vi "LVdouble connection.vi"() -> ()   [LabVIEW 2019]
doc: "This example performs a serial port write and a serial port read. The parameters set for the serial port must match the parameters of the connected instrument or device. The VISA Configure Serial Port VI sets the configuration parameters. The front panel displays the controls used to configure the basic parameters, such as baud rate, data bits, and parity. The VI passes the VISA resource name to other VIs that perform operations on that VISA resource. The VISA Write function sends a command to the serial device and the VISA Read function returns data based on the command. The VISA Close function then closes the reference to the serial device. It is important to close the reference; otherwise, further communication through that port might not be possible."
uses:
  Serial - Settings.ctl
  <vilib>/Utility/file.llb/Read Delimited Spreadsheet (DBL).vi
  <vilib>/Instr/_visa.llb/VISA Configure Serial Port (Instr).vi
panel:
  in  "Nominal Load Motor Torque":dbl=198.0
  out "Error Out":errorcluster={"status"=FALSE, "code"=1073676294, "source"="Event Code: 1073676294\r\nVISA Read in Read_Speed_Ref_1_21200.vi->LVdouble connection.vi\r\n-----------------------------------\nEvent Code: 1073676294\r\nVISA Read in Read_torque_Ref_1_21200.vi->LVdouble connection.vi\r\n-----------------------------------\n"}
  out "speed of the car km/h":dbl(knob)=0.002696450428155059 scale=0.0..10.0
  out "Execution time":u32(graph)=1000
  out "x-y 2":sgl
  out "String out":string
  out "read buffer 13":string
  out "read buffer 12":string
  out "read buffer 11":string
  out "read buffer 10":string
  out "read buffer 9":string
  out "read buffer 8":string
  out "read buffer 7":string
  out "Torque_Ref_readings":sgl(graph)
  in  "test_torque_setpoints":path=path "C:/Users/arda/Documents/GitHub/labviewtestbench/torque sp/simplified.txt"
  out "Power(kW)_PMSM":sgl(graph)=-5.360817e-06
  out "I_D":sgl(graph)=-0.16567513
  out "I_Q":sgl(graph)=-0.5964305
  out "I_PMSM":sgl(graph)
  out "Estimated Torque_PMSM":sgl(graph)=-0.5964305
  out "Read RPM-PMSM":dbl(graph)=-0.02861022762954235
  in  "data logging":bool=TRUE
  out "Serial Settings:Wire Mode 2":i8(ring)=-128 items=["Unknown"=-1, "RS485/Wire4"=0, "RS485/Wire2-EchoDTR"=1, "RS485/Wire2-CtrlDTR"=2, "RS485/Wire2-Auto"=3, "RS232/DTE"=-128, "RS232/DCE"=-127, "RS232/Auto"=-126]
  in  "timeout (10sec) 2":u32=10000
  in  "Enable Termination\nChar (T) 2":bool
  in  "Serial Settings 2":T1={"baud rate"=38400, "data bits"=8, "parity"=enum."Even", "stop bits"=10, "flow control"=0} {"flow control" items=["None"=0, "XON/XOFF"=1, "RTS/CTS"=2, "DTR/DSR"=4]; "stop bits" items=["1.0"=10, "1.5"=15, "2.0"=20]; "data bits" min=5 max=8 step=1; "baud rate" items=["75"=75, "110"=110, "134"=134, "150"=150, "300"=300, "600"=600, "1200"=1200, "1800"=1800, "2400"=2400, "4800"=4800, "9600"=7200, "19600"=9600, "14400"=14400, "19200"=19200, "28800"=28800, "38400"=38400, "56000"=56000, "57600"=57600, "115200"=115200, "128000"=128000, "230400"=230400]}
  in  "Hub Motor":refnum<visa-resource-name>="COM4"
  out "Torque Setpoints":dbl(graph)=4.4291015078268256e-09
  in  "Name your log file:":string="24_01_2020_low_cycle_100sec_on_inductionmotor"
  out "Speed Reference":sgl(graph)
  out "Speed Ref in 21202":string
  out "Floating Point 5":sgl
  out "Speed Ref in 21201":string
  in  "write buffer 5":string="\u0002\u0003RÑ\u0000\u0002„¹"
  out "Floating Point 4":sgl
  out "Speed Ref in 21201":string
  in  "write buffer 4":string="\u0002\u0003RÐ\u0000\u0002Õy"
  in  "write buffer 3":string="\u0002\u0003I<\u0000\u0002\u0012h"
  out "read buffer 6":string
  out "read buffer 5":string
  out "read buffer 4":string
  out "read buffer 3":string
  out "read buffer 2":string
  out "read buffer":string
  in  "write buffer 2":string="\u0002\u0003RÏ\u0000\u0002ä¿"
  in  "write buffer":string="\u0002\u0010RÏ\u0000\u0002\u0004\u0000\u0000@ d "
  out "Answer to Write Command":string
  out "Floating Point 3":sgl=5.00679
  out "Speed Ref in 21200":string
  out "Floating Point 2":sgl=0.14305113
  out "Speed Ref in Monitor":string
  out "I_D_IM":sgl(graph)=100.81332
  out "I_q_IM":sgl(graph)=-0.8283757
  out "Power(kW)_IM":sgl(graph)=-0.00012096913
  out "Current(I)_IM":sgl(graph)=100.730484
  in  "RPM and time setpoint file":path=path "C:/Users/arda/Documents/GitHub/labviewtestbench/RPM_setpointfile/ramp(1hz)_lowcycle.txt"
  in  "Tyre Diameter(m)":sgl=0.5
  out "Measured RPM_IM":sgl(graph)=0.028610228
  in  "Enum":T2(ring)=enum."Default"
  in  "Continuous Connection(Def:ON)":bool=TRUE
  out "Estimated Torque_IM":sgl(graph)=-4.347938
  in  "Finish session(Def:Off/False)":bool
  in  "Connectivity Check (Def:Off)":bool
  in  "timeout (10sec)":u32=10000
  out "connection check":u8[](array[numeric])=[0, 0, 0, 2]
  in  "Enable Termination\nChar (T)":bool
  in  "connection_verification":string="\u0002\u0003Fm\u0000\u0002@­"
  out "Serial Settings:Wire Mode":i8(ring)=-128 items=["Unknown"=-1, "RS485/Wire4"=0, "RS485/Wire2-EchoDTR"=1, "RS485/Wire2-CtrlDTR"=2, "RS485/Wire2-Auto"=3, "RS232/DTE"=-128, "RS232/DCE"=-127, "RS232/Auto"=-126]
  in  "Serial Settings":T1={"baud rate"=38400, "data bits"=8, "parity"=enum."Even", "stop bits"=10, "flow control"=0} {"flow control" items=["None"=0, "XON/XOFF"=1, "RTS/CTS"=2, "DTR/DSR"=4]; "stop bits" items=["1.0"=10, "1.5"=15, "2.0"=20]; "data bits" min=5 max=8 step=1; "baud rate" items=["75"=75, "110"=110, "134"=134, "150"=150, "300"=300, "600"=600, "1200"=1200, "1800"=1800, "2400"=2400, "4800"=4800, "9600"=7200, "19600"=9600, "14400"=14400, "19200"=19200, "28800"=28800, "38400"=38400, "56000"=56000, "57600"=57600, "115200"=115200, "128000"=128000, "230400"=230400]}
  in  "Induction Motor":refnum<visa-resource-name>="COM3"
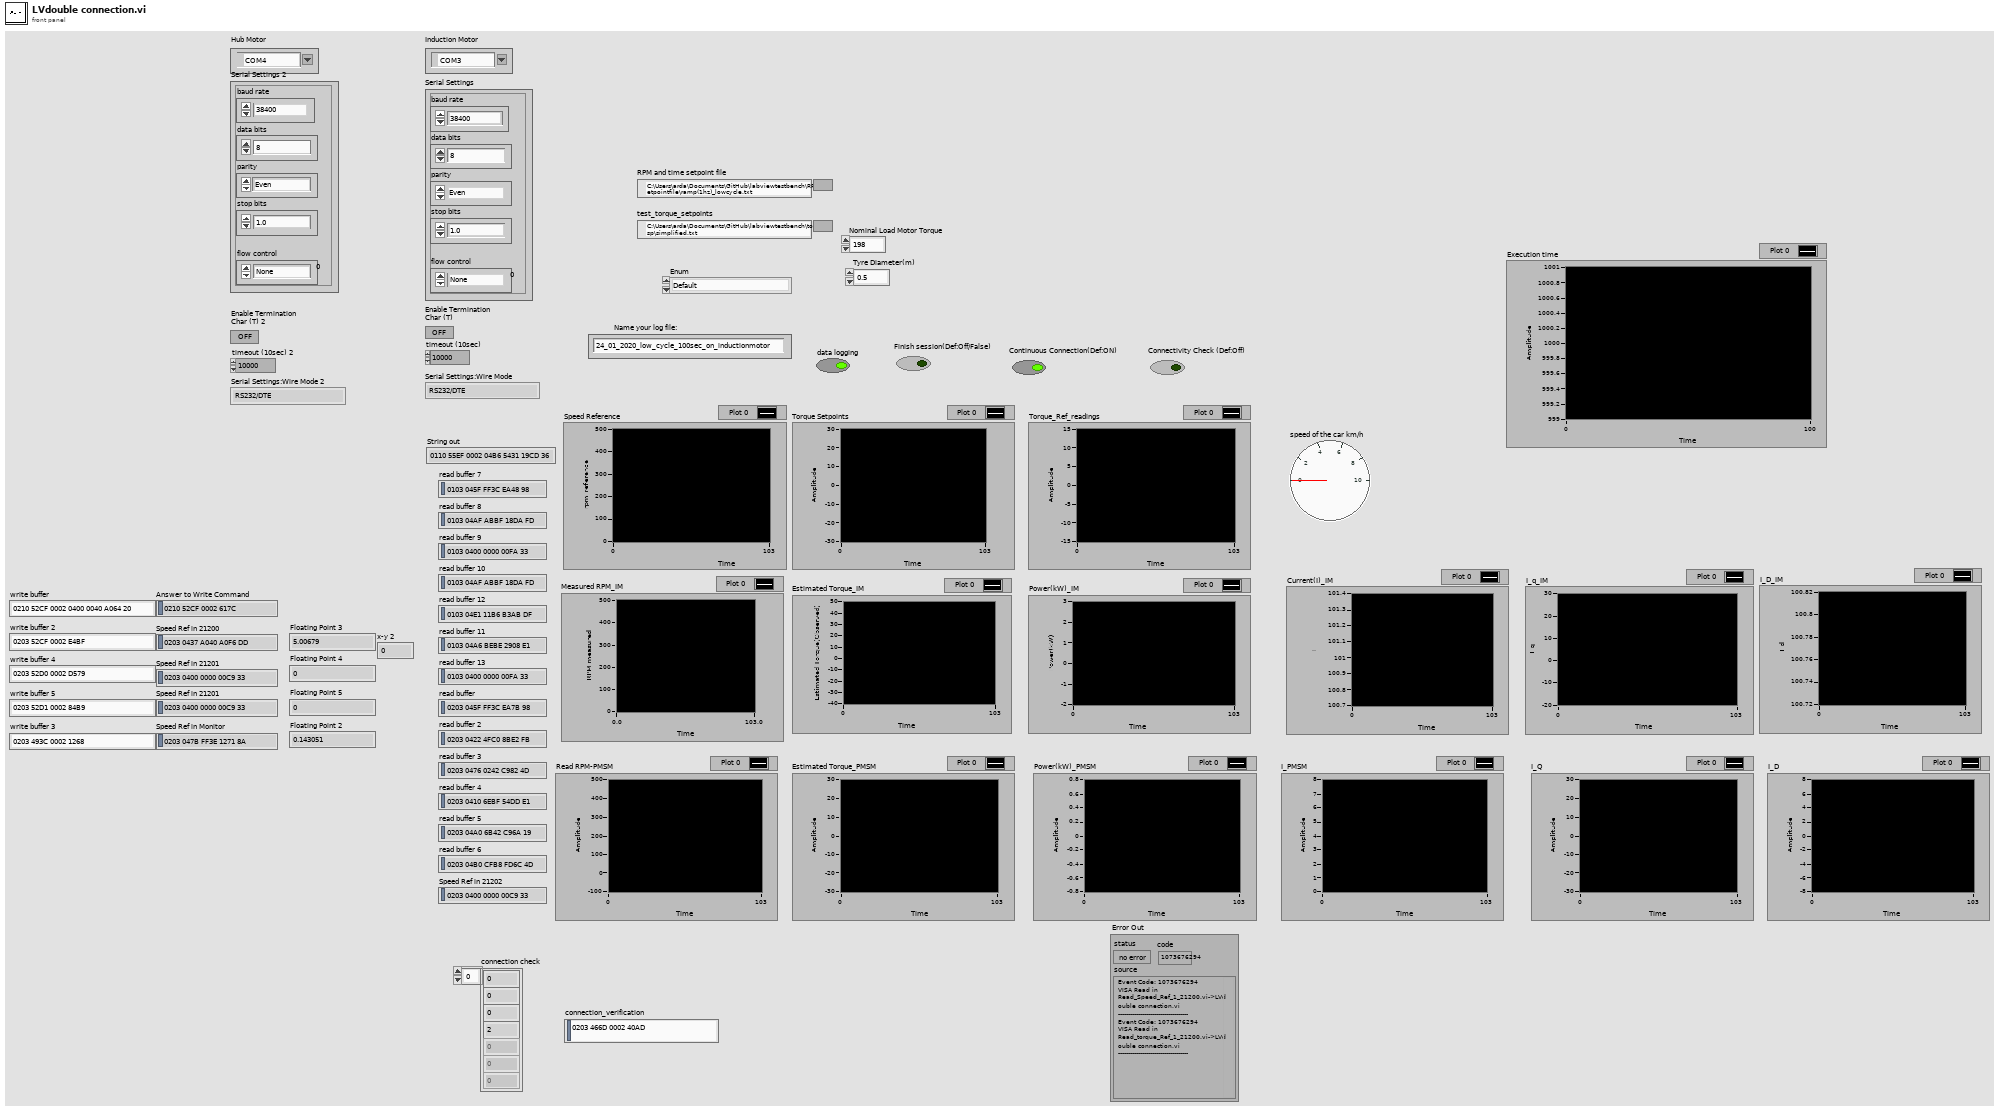
[diagram p1: front panel]
types:
  T1 = typedef "Serial - Settings.ctl" = cluster{"baud rate":u32, "data bits":u16, "parity":enum16{"None", "Odd", "Even", "Mark", "Space"}, "stop bits":u16, "flow control":u16}
  T2 = enum16{"Single Signal Trials", "Default", "Alarm Reset", "Write Save Command", "Drive Reset"}
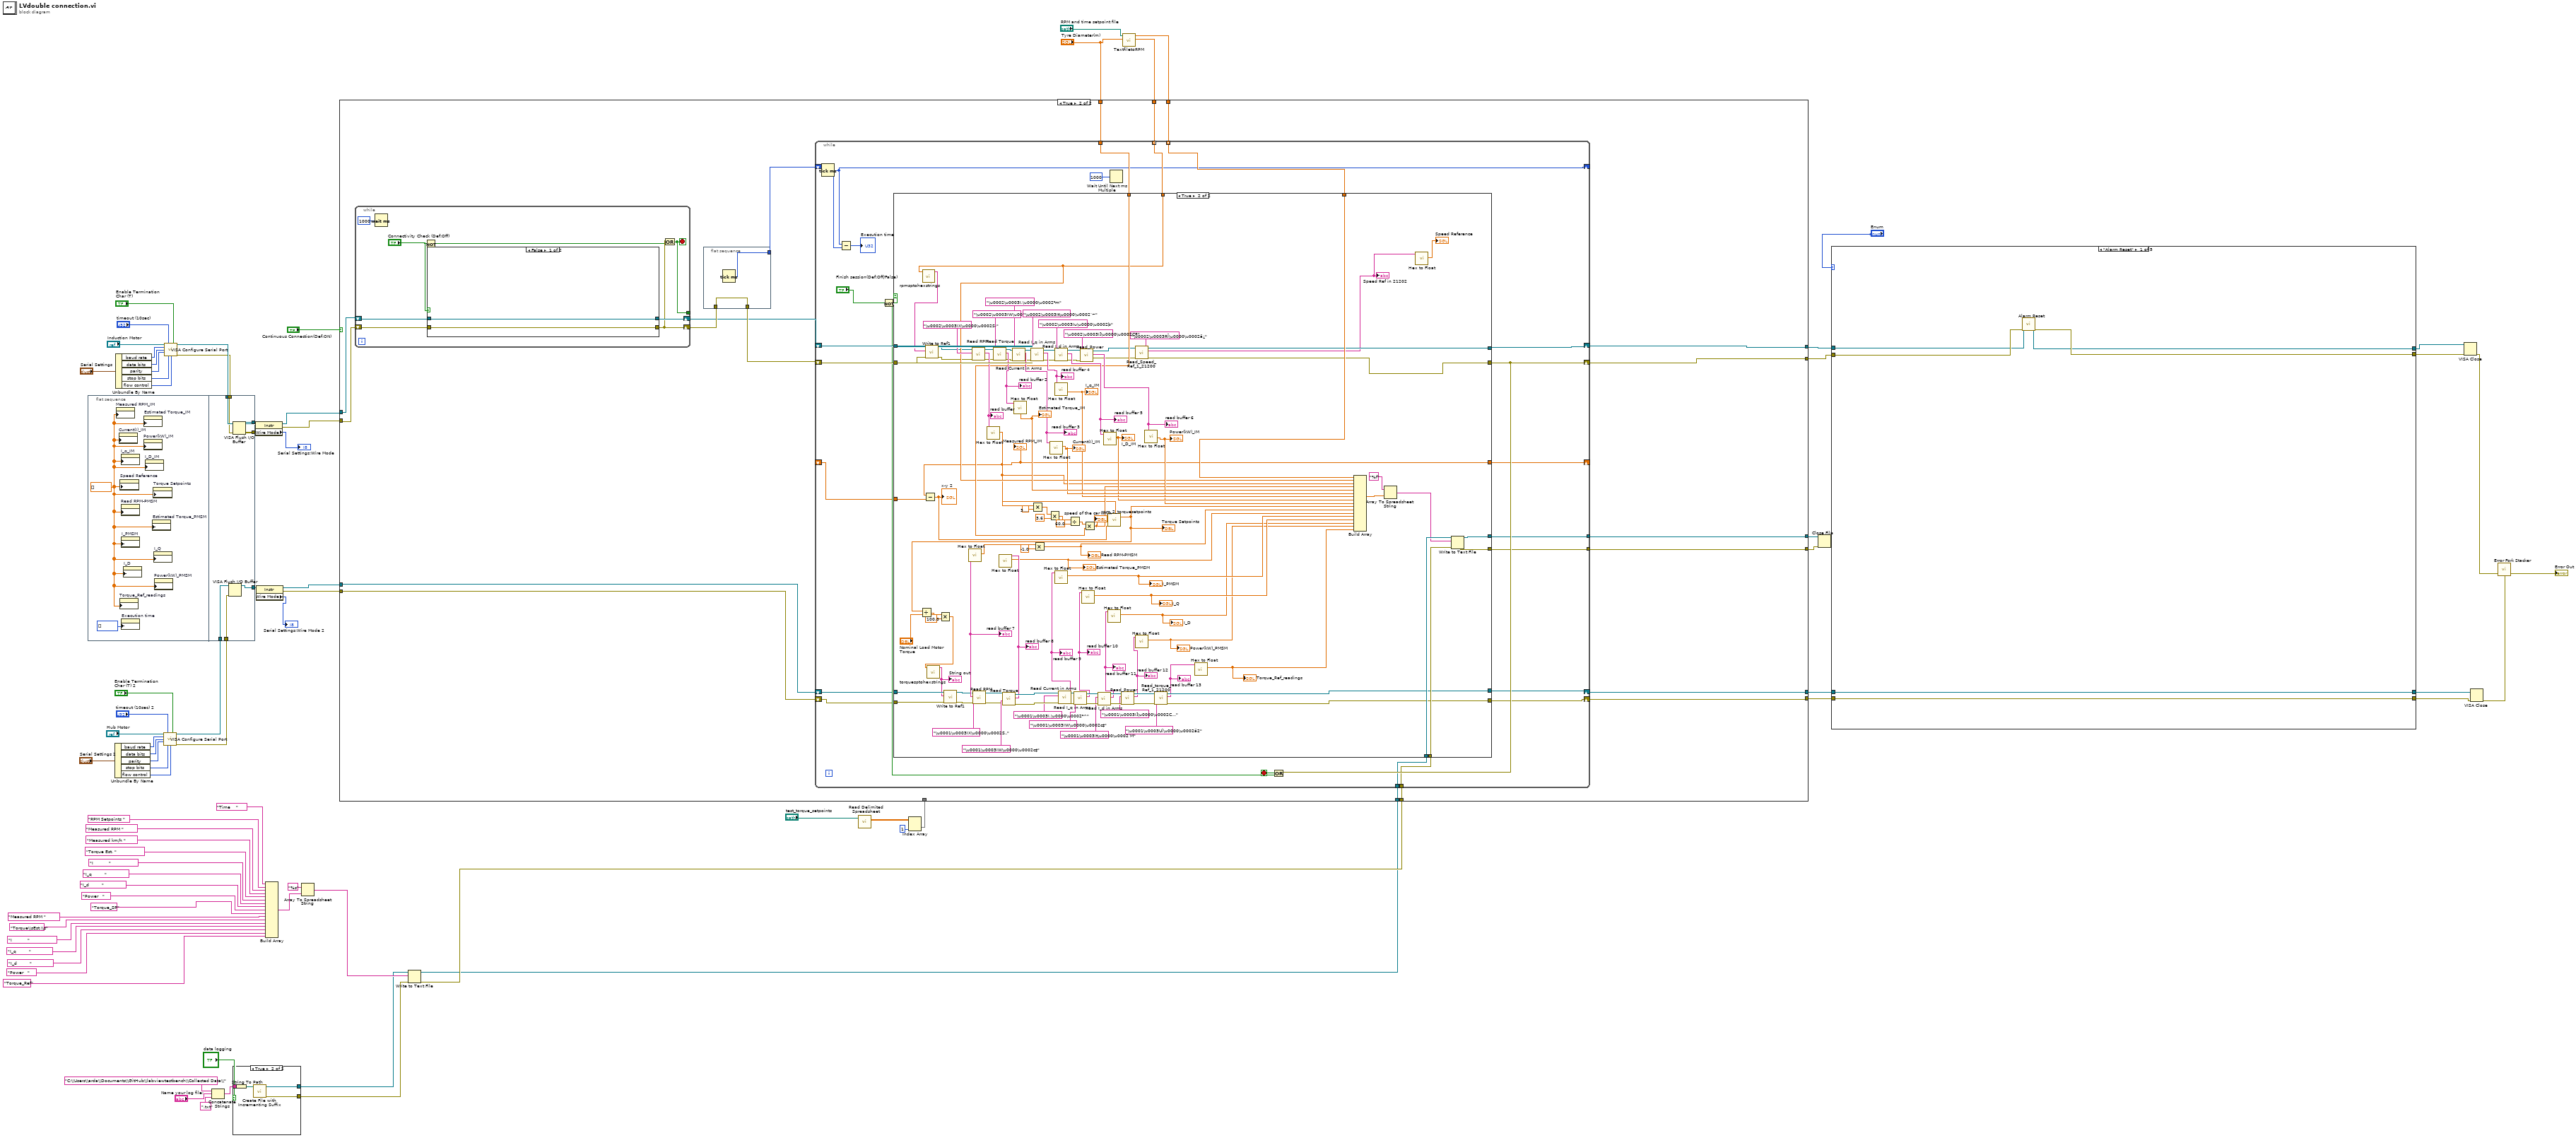
[diagram p0: block diagram]
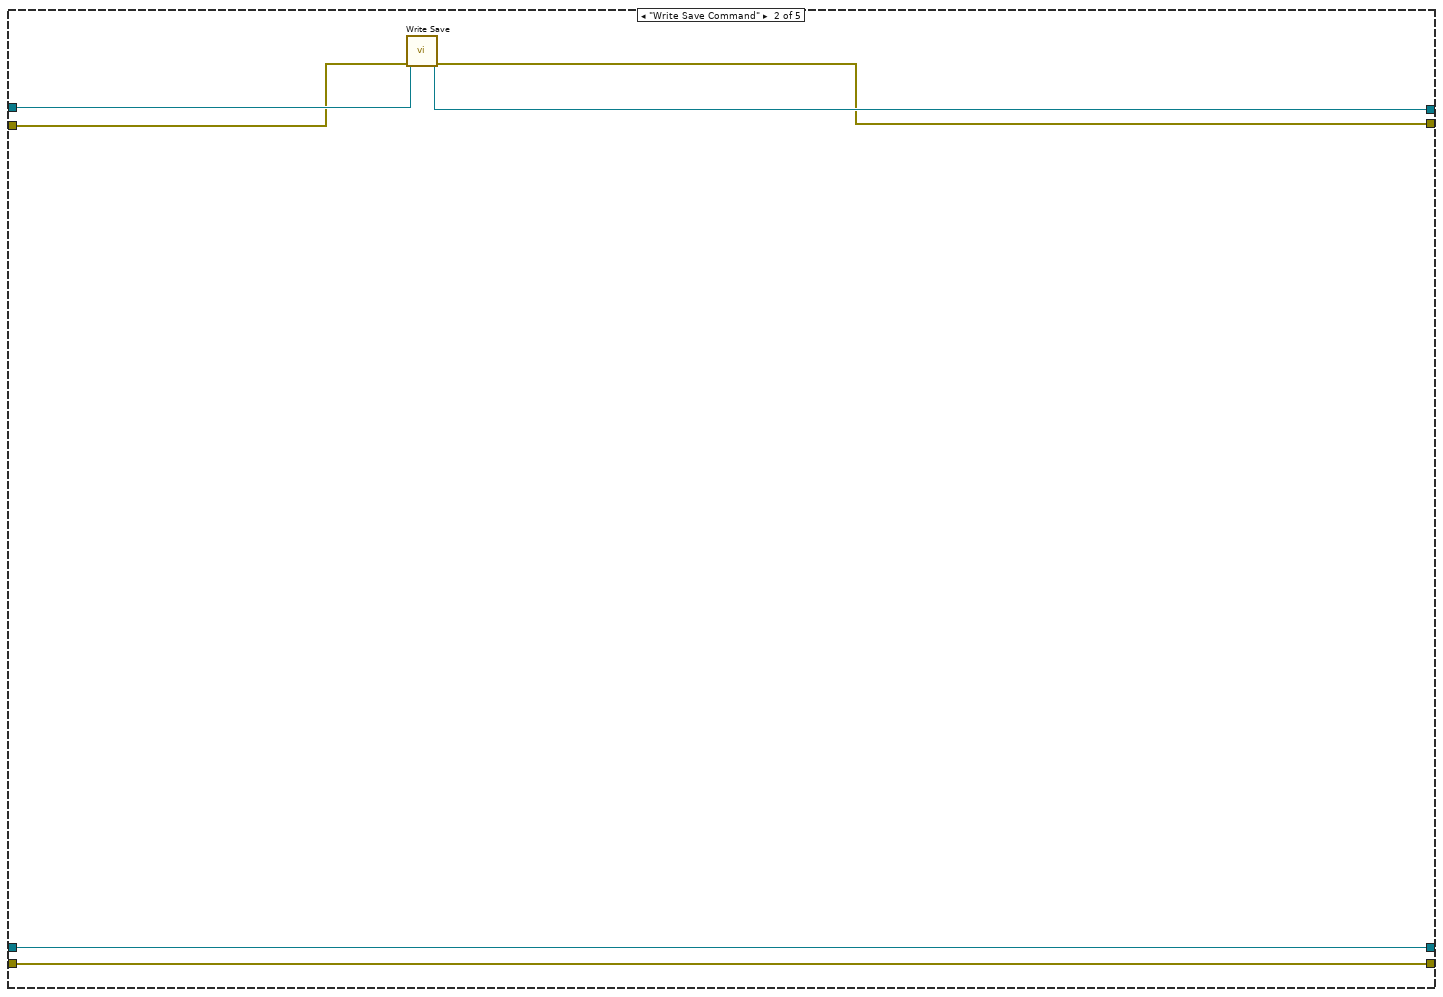
[diagram p3: hidden frame]
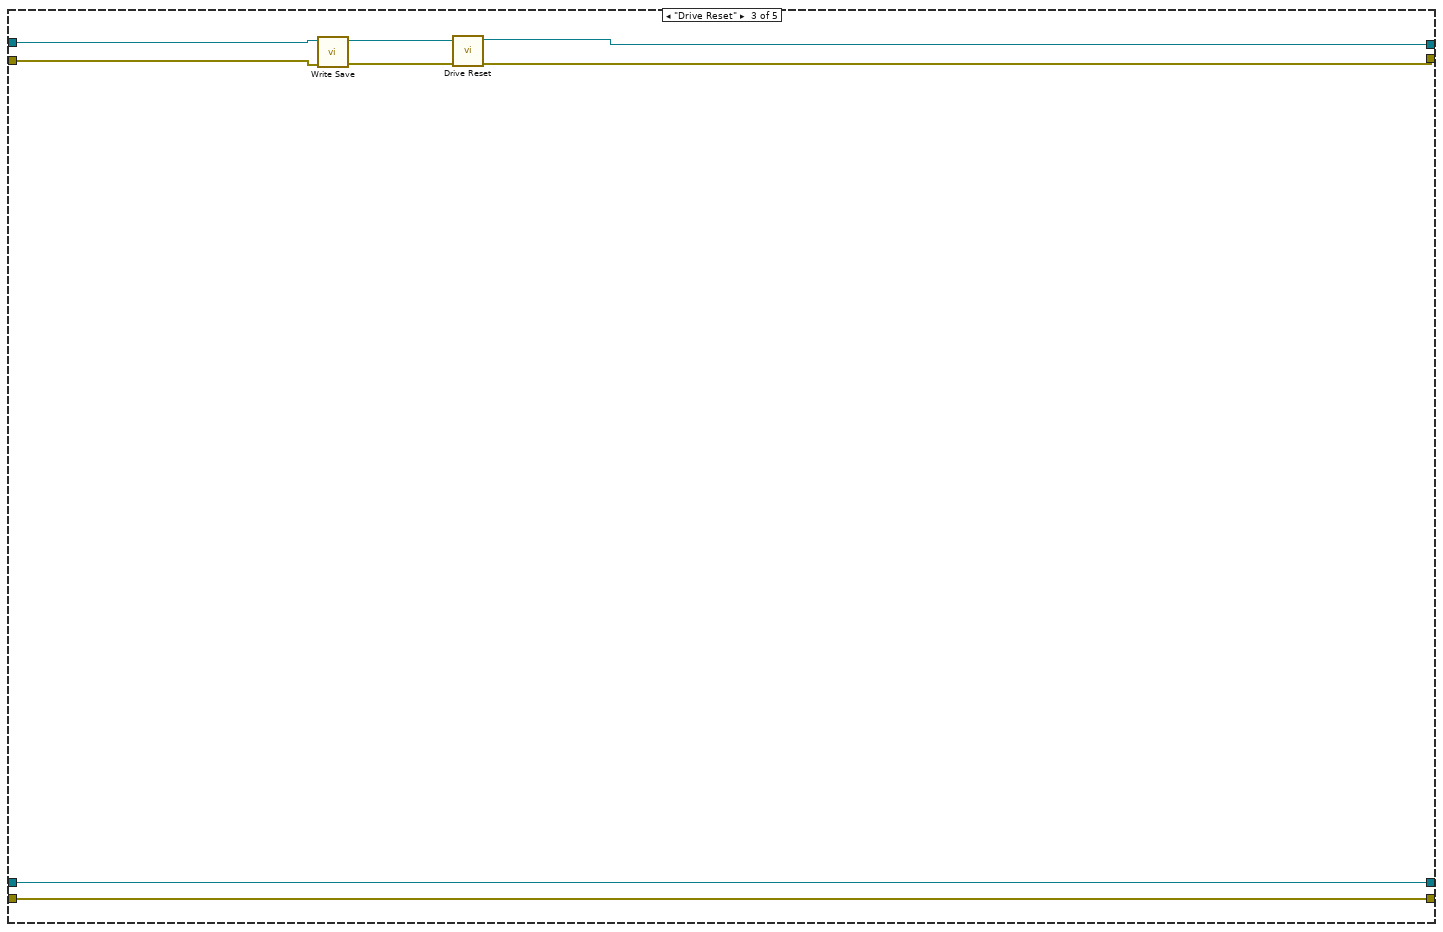
[diagram p4: hidden frame]
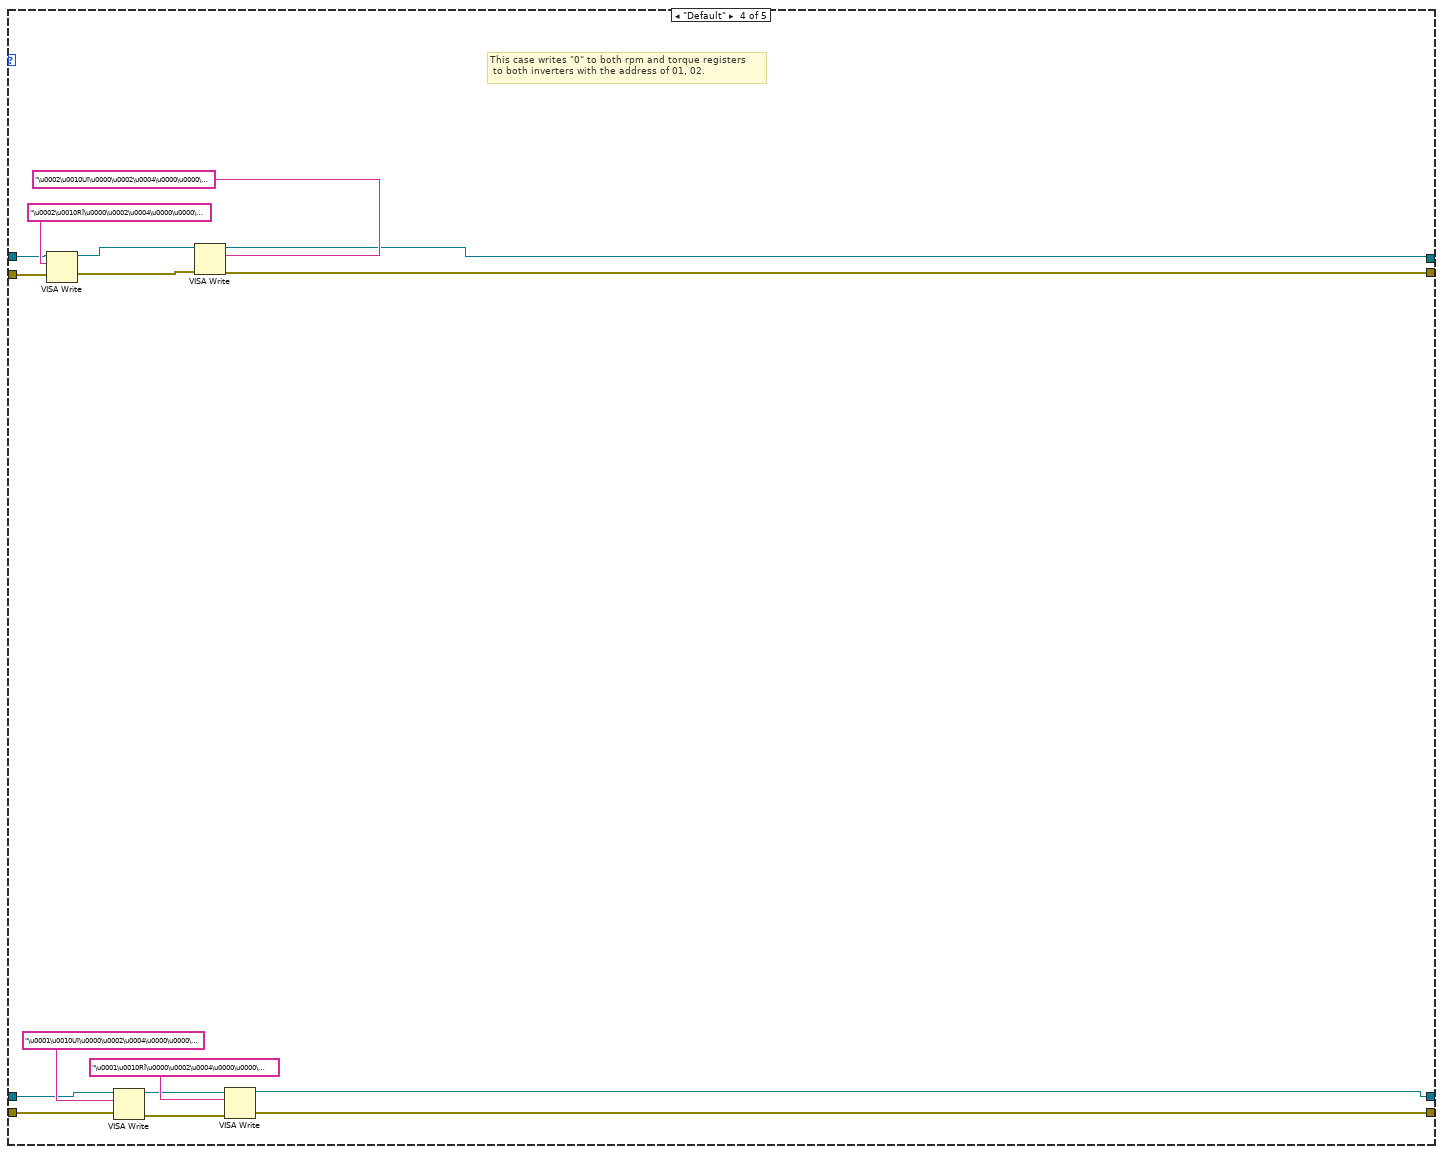
[diagram p5: hidden frame]
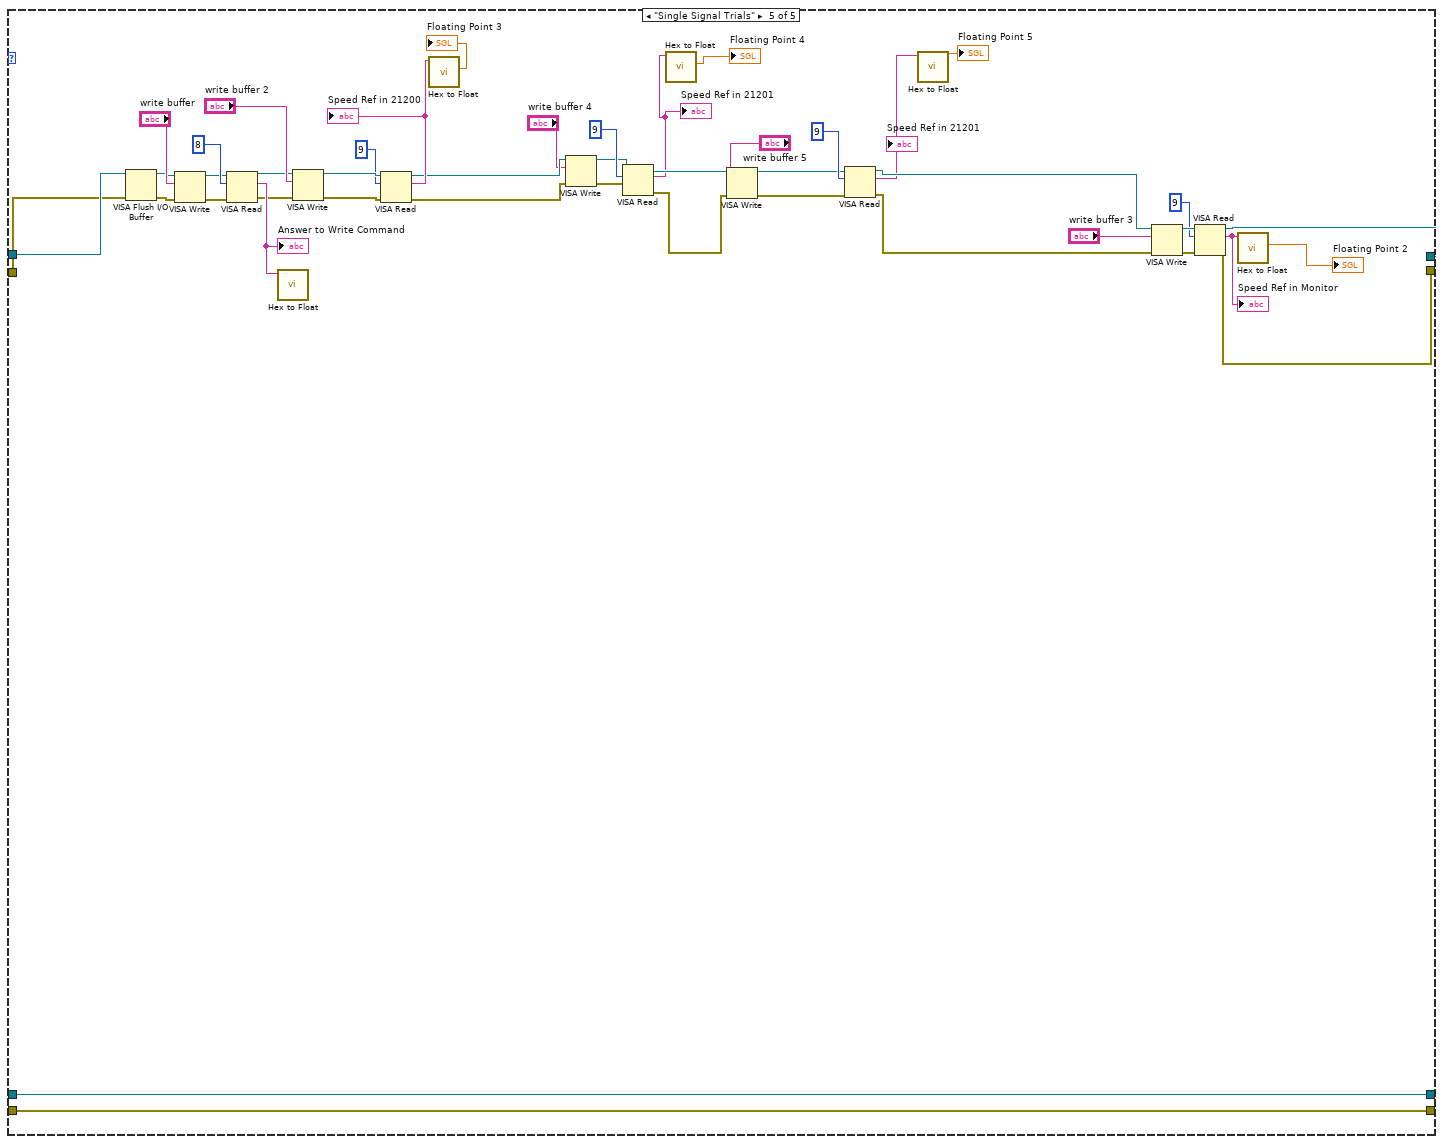
[diagram p6: hidden frame]
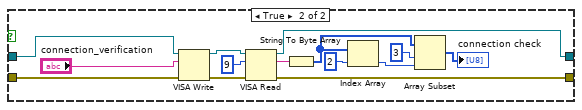
[diagram p8: hidden frame]
diagram:
  n1 = flat-sequence {
    tunnel: [w92] -> w82
    tunnel: [w91] -> w81
    tunnel: w80 -> [w90]
    tunnel: w79 -> [w89]
    tunnel: w43 -> [w88]
    tunnel: w42 -> [w87]
    tunnel: [w86] -> w41
    frame #0 {
      w85 = sgl[] [] ("History Data")
      n2 = property on="Measured RPM_IM" class="WFChart (strict)"("History Data"=w85) -> ()  [unwired: 2 in, 2 out]
      n3 = property on="Current(I)_IM" class="WFChart (strict)"("History Data"=w85) -> ()  [unwired: 2 in, 2 out]
      n4 = property on="Torque_Ref_readings" class="WFChart (strict)"("History Data"=w85) -> ()  [unwired: 2 in, 2 out]
      n5 = property on="Speed Reference" class="WFChart (strict)"("History Data"=w85) -> ()  [unwired: 2 in, 2 out]
      n6 = property on="I_q_IM" class="WFChart (strict)"("History Data"=w85) -> ()  [unwired: 2 in, 2 out]
      n7 = property on="Read RPM-PMSM" class="WFChart (strict)"("History Data"=w85) -> ()  [unwired: 2 in, 2 out]
      n8 = property on="I_PMSM" class="WFChart (strict)"("History Data"=w85) -> ()  [unwired: 2 in, 2 out]
      n9 = property on="Execution time" class="WFChart (strict)"("History Data"=u32[] []) -> ()  [unwired: 2 in, 2 out]
      n10 = property on="I_D" class="WFChart (strict)"("History Data"=w85) -> ()  [unwired: 2 in, 2 out]
      n11 = property on="Power(kW)_IM" class="WFChart (strict)"("History Data"=w85) -> ()  [unwired: 2 in, 2 out]
      n12 = property on="Estimated Torque_IM" class="WFChart (strict)"("History Data"=w85) -> ()  [unwired: 2 in, 2 out]
      n13 = property on="I_D_IM" class="WFChart (strict)"("History Data"=w85) -> ()  [unwired: 2 in, 2 out]
      n14 = property on="Estimated Torque_PMSM" class="WFChart (strict)"("History Data"=w85) -> ()  [unwired: 2 in, 2 out]
      n15 = property on="Torque Setpoints" class="WFChart (strict)"("History Data"=w85) -> ()  [unwired: 2 in, 2 out]
      n16 = property on="I_Q" class="WFChart (strict)"("History Data"=w85) -> ()  [unwired: 2 in, 2 out]
      n17 = property on="Power(kW)_PMSM" class="WFChart (strict)"("History Data"=w85) -> ()  [unwired: 2 in, 2 out]
    }
    frame #1 {
      n18 = VISA Flush I/O Buffer(VISA resource name=w88, error in (no error)=w87) -> (VISA resource name out=w86:refnum<visa-resource-name>)  [unwired: 1 in, 1 out]
      n19 = VISA Flush I/O Buffer(VISA resource name=w90, error in (no error)=w89) -> (VISA resource name out=w91:refnum<visa-resource-name>, error out=w92:errorcluster)  [unwired: 1 in]
    }
  }
  n20 = Unbundle By Name("Serial Settings 2") -> ("baud rate"=w10:u32, "data bits"=w14:u16, "parity"=w13:enum16{"None", "Odd", "Even", "Mark", "Space"}, "stop bits"=w12:u16, "flow control"=w11:u16)
  n21 = Unbundle By Name("Serial Settings") -> ("baud rate"=w19:u32, "data bits"=w23:u16, "parity"=w22:enum16{"None", "Odd", "Even", "Mark", "Space"}, "stop bits"=w21:u16, "flow control"=w20:u16)
  n22 = call-poly "VISA Configure Serial Port"("VISA resource name"="Hub Motor", "timeout (10sec)"="timeout (10sec) 2", "Enable Termination\nChar (T)"="Enable Termination\nChar (T) 2", "baud rate (9600)"=w10, "data bits (8)"=w14, "parity (0:none)"=w13, "stop bits (10: 1 bit)"=w12, "flow control (0:none)"=w11) -> ("VISA resource name out"=w43:refnum<visa-resource-name>, "error out"=w42:errorcluster)  [unwired: 1 in, 5 out]
  n23 = call-poly "VISA Configure Serial Port"("VISA resource name"="Induction Motor", "timeout (10sec)"="timeout (10sec)", "Enable Termination\nChar (T)"="Enable Termination\nChar (T)", "baud rate (9600)"=w19, "data bits (8)"=w23, "parity (0:none)"=w22, "stop bits (10: 1 bit)"=w21, "flow control (0:none)"=w20) -> ("VISA resource name out"=w80:refnum<visa-resource-name>, "error out"=w79:errorcluster)  [unwired: 1 in, 5 out]
  n24 = Concatenate Strings("C:\\Users\\arda\\Documents\\GitHub\\labviewtestbench\\Collected Data\\" ("string"), "Name your log file:", ".txt") -> (w63:string)
  n25 = case shown="True" "data logging" {
    tunnel: w63 -> [_ w96]
    tunnel: [_ w94] -> w59
    tunnel: [_ w93] -> w58
    frame False {
    }
    frame True {
      n26 = String To Path(string=w96) -> (path=w95:path)
      n27 = call <vilib>:"Create File with Incrementing Suffix.vi"("file path"=w95) -> ("error out"=w93:errorcluster, "refnum out"=w94:refnum<file>)  [unwired: 8 in, 1 out]
    }
  }
  n28 = property class="Instr"(reference=w81, error in=w82) -> (reference out=w77:refnum<visa-resource-name>, error out=w78:errorcluster, "Wire Mode"=→"Serial Settings:Wire Mode":i16)
  n29 = property class="Instr"(reference=w41) -> (reference out=w39:refnum<visa-resource-name>, error out=w38:errorcluster, "Wire Mode"=→"Serial Settings:Wire Mode 2":i16)  [unwired: 1 in]
  n30 = Build Array("Time    " ("element"), "RPM Setpoints ", "Measured RPM ", "Measured km/h ", "Torque Est. ", "I           " ("element"), "I_q         " ("element"), "I_d         " ("element"), "Power   " ("element"), "Torque_SP" ("element"), "Measured RPM ", "Torque\\sEst.\\s" ("element"), "I           " ("element"), "I_q         " ("element"), "I_d         " ("element"), "Power   " ("element"), "Torque_Ref" ("element")) -> (w66:string[])
  n31 = Array To Spreadsheet String(array=w66, 3:"%s" ("format string")) -> (spreadsheet string=w64:string)  [unwired: 1 in]
  n32 = Write to Text File(file (use dialog)=w59, text=w64, error in=w58) -> (refnum out=w51:refnum<file>, error out=w52:errorcluster)  [unwired: 1 in, 1 out]
  n33 = call-poly <vilib>:"Read Delimited Spreadsheet.vi"("file path (dialog if empty)"="test_torque_setpoints") -> ("all rows"=w29:dbl[][])  [unwired: 9 in, 5 out]
  n34 = Index Array(array=w29, index (col)=1 ("disabled index (col)")) -> (element=w27:dbl[])  [unwired: 1 in]
  n35 = call "TextfiletoRPM.vi"("Tyre Diameter(m)"="Tyre Diameter(m)", "file path (dialog if empty)"="RPM and time setpoint file") -> ("Array"=w71:dbl[], "time_sp"=w50:sgl[])  [unwired: 8 in]
  n36 = case shown="True" "Continuous Connection(Def:ON)" {
    tunnel: w78 -> [w101 w107]
    tunnel: w77 -> [w102 w121]
    tunnel: [w102 w120] -> w76
    tunnel: w71 -> [_ w119]
    tunnel: [w101 w118] -> w69
    tunnel: w51 -> [w99 w117]
    tunnel: w52 -> [w100 w116]
    tunnel: [w99 w115] -> w68
    tunnel: [w100 w114] -> w67
    tunnel: w50 -> [_ w113]
    tunnel: "Tyre Diameter(m)" -> [_ w112]
    tunnel: w39 -> [w97 w106]
    tunnel: w38 -> [w98 w105]
    tunnel: [w97 w104] -> w7
    tunnel: [w98 w103] -> w6
    tunnel: w27 -> [_ _]
    frame False {
    }
    frame True {
      n37 = while {
        shift-right: [w131] -> w109
        shift-left: w121 -> [w130]
        shift-right: [w128] -> w111
        shift-left: w107 -> [w129]
        tunnel: [w124] -> _
        stop <- w124 stop-if-true
        n38 = Wait (ms)(milliseconds to wait=u32 1000) -> ()  [unwired: 1 out]
        n39 = Not(x="Connectivity Check (Def:Off)") -> (.not. x?=w125:bool)
        n40 = case shown="False" "Connectivity Check (Def:Off)" {
          tunnel: [w133 w147] -> w131
          tunnel: w130 -> [w133 w146]
          tunnel: w129 -> [w132 w145]
          tunnel: [w132 w144] -> w128
          frame False {
          }
          frame True {
            n41 = VISA Write(VISA resource name=w146, write buffer="connection_verification", error in (no error)=w145) -> (VISA resource name out=w143:refnum<visa-resource-name>, error out=w141:errorcluster)  [unwired: 1 out]
            n42 = VISA Read(VISA resource name=w143, byte count=u32 9, error in (no error)=w141) -> (VISA resource name out=w147:refnum<visa-resource-name>, read buffer=w135:string, error out=w144:errorcluster)  [unwired: 1 out]
            n43 = String To Byte Array(string=w135) -> (unsigned byte array=w139:u8[])
            n44 = Index Array(array=w139, index=2) -> (element=w136:u8)
            n45 = Array Subset(array=w139, index=3 ("length"), length=w136) -> (→"connection check":u8[])
          }
        }
        n46 = Or(x=w128, y=w125) -> (x .or. y?=w124:bool)
      }
      n47 = flat-sequence {
        tunnel: [w123] -> w110
        tunnel: w111 -> [w123]
        tunnel: [w122] -> w108
        frame #0 {
          n48 = Tick Count (ms)() -> (millisecond timer value=w122:u32)
        }
      }
      n49 = while {
        shift-right: [w169] -> w120
        shift-left: w109 -> [w171]
        shift-right: [w168] -> w118
        shift-left: w110 -> [w170]
        tunnel: w119 -> [w166] mode=indexing
        tunnel: w117 -> [w164]
        tunnel: w116 -> [w163]
        tunnel: [w162] -> w115
        tunnel: [w161] -> w114
        tunnel: w113 -> [w160] mode=indexing
        tunnel: w112 -> [w159]
        shift-right: [w155] -> _
        shift-left: w108 -> [w156]
        shift-right: [w151] -> w104
        shift-left: w106 -> [w153]
        shift-right: [w150] -> w103
        shift-left: w105 -> [w152]
        shift-right: [w149] -> _
        shift-left: _ -> [w148]
        stop <- w167 stop-if-true
        n50 = Tick Count (ms)() -> (millisecond timer value=w155:u32)
        n51 = Subtract(x=w155, y=w156) -> (x-y=→"Execution time":u32)
        n52 = Not(x="Finish session(Def:Off/False)") -> (.not. x?=w157:bool)
        n53 = case shown="True" w157 {
          tunnel: w171 -> [w178 w202]
          tunnel: w170 -> [w177 w201]
          tunnel: [w178 w228] -> w169
          tunnel: [w177 w226] -> w168
          tunnel: w166 -> [_ w229]
          tunnel: w164 -> [w176 w270]
          tunnel: w163 -> [w175 w269]
          tunnel: [w176 w268] -> w162
          tunnel: [w175 w267] -> w161
          tunnel: w160 -> [_ w258]
          tunnel: w159 -> [_ w257]
          tunnel: w153 -> [w173 w207]
          tunnel: w152 -> [w174 w206]
          tunnel: [w173 w231] -> w151
          tunnel: [w174 w230] -> w150
          tunnel: [w172 w187] -> w149
          tunnel: w148 -> [w172 w186]
          frame False {
          }
          frame True {
            n54 = call "rpmsptohexstrings.vi"("RPM value"=w229) -> ("String out"=w198:string)  [unwired: 10 in]
            n55 = call "Write to Ref1.vi"("error in (no error)"=w201, "String in"=w198, "VISA Refnum in"=w202) -> ("error out"=w199:errorcluster, "VISA Refnum out"=w200:refnum<visa-resource-name>)  [unwired: 6 in, 1 out]
            n56 = call "Read RPM.vi"("error in (no error)"=w199, "write buffer"="\u0002\u0003IX\u0000\u0002S·", "VISA resource name"=w200) -> ("error out"=w212:errorcluster, "read buffer"=w283:string, "VISA resource name out"=w256:refnum<visa-resource-name>)  [unwired: 6 in]
            "read buffer" <- w283
            n57 = call "Hex to Float.vi"("read buffer in"=w283) -> ("Floating Point"=w187:sgl)  [unwired: 9 in, 1 out]
            "Measured RPM_IM" <- w187
            n58 = Subtract(x=w187, y=w186) -> (x-y=w185:sgl)
            "x-y 2" <- w185
            n59 = call "Read Torque.vi"("error in (no error)"=w212, "Real Torque"="\u0002\u0003IW\u0000\u0002c´", "VISA Refnum in"=w256) -> ("error out"=w248:errorcluster, "read buffer"=w284:string, "VISA Refnum out"=w255:refnum<visa-resource-name>)  [unwired: 6 in]
            "read buffer 2" <- w284
            n60 = call "Read Current in Arms.vi"("error in (no error)"=w248, "write buffer"="\u0002\u0003I.\u0000\u0002²m", "VISA Refnum in"=w255) -> ("error out"=w249:errorcluster, "read buffer"=w281:string, "VISA Refnum out"=w254:refnum<visa-resource-name>)  [unwired: 6 in]
            "read buffer 3" <- w281
            n61 = call "Hex to Float.vi"("read buffer in"=w284) -> ("Floating Point"=w277:sgl)  [unwired: 9 in, 1 out]
            "Estimated Torque_IM" <- w277
            n62 = call "Read I_q in Arms.vi"("error in (no error)"=w249, "write buffer 2"="\u0002\u0003It\u0000\u0002’~", "VISA Refnum in"=w254) -> ("error out"=w250:errorcluster, "read buffer"=w280:string, "VISA Refnum out"=w253:refnum<visa-resource-name>)  [unwired: 6 in]
            "read buffer 4" <- w280
            n63 = Multiply(x=w187, y=3.141592653589793) -> (x*y=w264:dbl)
            n64 = Multiply(x=w264, y=3.6) -> (x*y=w262:dbl)
            n65 = call "Hex to Float.vi"("read buffer in"=w281) -> ("Floating Point"=w276:sgl)  [unwired: 9 in, 1 out]
            "Current(I)_IM" <- w276
            n66 = call "Read I_d in Arms.vi"("error in (no error)"=w250, "write buffer"="\u0002\u0003Iu\u0000\u0002þ", "VISA Refnum in"=w253) -> ("error out"=w251:errorcluster, "read buffer"=w279:string, "VISA Refnum out"=w252:refnum<visa-resource-name>)  [unwired: 6 in]
            "read buffer 5" <- w279
            n67 = call "Hex to Float.vi"("read buffer in"=w280) -> ("Floating Point"=w275:sgl)  [unwired: 9 in, 1 out]
            "I_q_IM" <- w275
            n68 = Divide(x=w262, y=60.0) -> (x/y=w260:dbl)
            n69 = call "Read_Power.vi"("error in (no error)"=w251, "write buffer"="\u0002\u0003I]\u0000\u0002C¶", "VISA Refnum in"=w252) -> ("error out"=w196:errorcluster, "read buffer"=w282:string, "VISA Refnum out"=w197:refnum<visa-resource-name>)  [unwired: 6 in]
            "read buffer 6" <- w282
            n70 = Multiply(x=w260, y=w257) -> (x*y=w259:dbl)
            "speed of the car km/h" <- w259
            n71 = call "Hex to Float.vi"("read buffer in"=w279) -> ("Floating Point"=w274:sgl)  [unwired: 9 in, 1 out]
            "I_D_IM" <- w274
            n72 = call "rpm_2_torquesetpoints.vi"("derivative"=w185, "RPM"=w187) -> ("Torque Setpoints_graph_percentage"=w184:dbl)  [unwired: 10 in, 7 out]
            "Torque Setpoints" <- w184
            n73 = Divide(x=w184, y="Nominal Load Motor Torque") -> (x/y=w182:dbl)
            n74 = Multiply(x=w182, y=100.0) -> (x*y=w180:dbl)
            n75 = call "torquesptohexstrings.vi"("Torque Value"=w180) -> ("String out"=w188:string)  [unwired: 10 in]
            "String out" <- w188
            n76 = call "Write to Ref1.vi"("error in (no error)"=w206, "String in"=w188, "VISA Refnum in"=w207) -> ("error out"=w204:errorcluster, "VISA Refnum out"=w205:refnum<visa-resource-name>)  [unwired: 6 in, 1 out]
            n77 = call "Read RPM.vi"("error in (no error)"=w204, "write buffer"="\u0001\u0003IX\u0000\u0002S„", "VISA resource name"=w205) -> ("error out"=w211:errorcluster, "read buffer"=w223:string, "VISA resource name out"=w247:refnum<visa-resource-name>)  [unwired: 6 in]
            "read buffer 7" <- w223
            n78 = call "Hex to Float.vi"("read buffer in"=w223) -> ("Floating Point"=w209:sgl)  [unwired: 9 in, 1 out]
            n79 = call "Read Torque.vi"("error in (no error)"=w211, "Real Torque"="\u0001\u0003IW\u0000\u0002c‡", "VISA Refnum in"=w247) -> ("error out"=w245:errorcluster, "read buffer"=w222:string, "VISA Refnum out"=w246:refnum<visa-resource-name>)  [unwired: 6 in]
            "read buffer 8" <- w222
            n80 = call "Hex to Float.vi"("read buffer in"=w222) -> ("Floating Point"=w221:sgl)  [unwired: 9 in, 1 out]
            "Estimated Torque_PMSM" <- w221
            n81 = Multiply(x=w209, y=-1.0) -> (x*y=w208:dbl)
            "Read RPM-PMSM" <- w208
            n82 = call "Read Current in Arms.vi"("error in (no error)"=w245, "write buffer"="\u0001\u0003I.\u0000\u0002²^", "VISA Refnum in"=w246) -> ("error out"=w243:errorcluster, "read buffer"=w220:string, "VISA Refnum out"=w244:refnum<visa-resource-name>)  [unwired: 6 in]
            "read buffer 9" <- w220
            n83 = call "Hex to Float.vi"("read buffer in"=w220) -> ("Floating Point"=w219:sgl)  [unwired: 9 in, 1 out]
            "I_PMSM" <- w219
            n84 = call "Read I_q in Arms.vi"("error in (no error)"=w243, "write buffer 2"="\u0001\u0003IW\u0000\u0002c‡", "VISA Refnum in"=w244) -> ("error out"=w241:errorcluster, "read buffer"=w218:string, "VISA Refnum out"=w242:refnum<visa-resource-name>)  [unwired: 6 in]
            "read buffer 10" <- w218
            n85 = call "Hex to Float.vi"("read buffer in"=w218) -> ("Floating Point"=w217:sgl)  [unwired: 9 in, 1 out]
            "I_Q" <- w217
            n86 = call "Read I_d in Arms.vi"("error in (no error)"=w241, "write buffer"="\u0001\u0003It\u0000\u0002’M", "VISA Refnum in"=w242) -> ("error out"=w239:errorcluster, "read buffer"=w216:string, "VISA Refnum out"=w240:refnum<visa-resource-name>)  [unwired: 6 in]
            "read buffer 11" <- w216
            n87 = call "Hex to Float.vi"("read buffer in"=w216) -> ("Floating Point"=w215:sgl)  [unwired: 9 in, 1 out]
            "I_D" <- w215
            n88 = call "Read_Power.vi"("error in (no error)"=w239, "write buffer"="\u0001\u0003I]\u0000\u0002C…", "VISA Refnum in"=w240) -> ("error out"=w224:errorcluster, "read buffer"=w214:string, "VISA Refnum out"=w225:refnum<visa-resource-name>)  [unwired: 6 in]
            "read buffer 12" <- w214
            n89 = call "Read_Speed_Ref_1_21200.vi"("error in (no error)"=w196, "write buffer 7"="\u0002\u0003RÏ\u0000\u0002ä¿", "VISA Refnum in"=w197) -> ("error out"=w226:errorcluster, "read buffer"=w227:string, "VISA Refnum out"=w228:refnum<visa-resource-name>)  [unwired: 6 in]
            "Speed Ref in 21202" <- w227
            n90 = call "Hex to Float.vi"("read buffer in"=w214) -> ("Floating Point"=w213:sgl)  [unwired: 9 in, 1 out]
            "Power(kW)_PMSM" <- w213
            n91 = call "Hex to Float.vi"("read buffer in"=w282) -> ("Floating Point"=w273:sgl)  [unwired: 9 in, 1 out]
            "Power(kW)_IM" <- w273
            n92 = call "Read_torque_Ref_1_21200.vi"("error in (no error)"=w224, "write buffer 7"="\u0001\u0003Uï\u0000\u0002ä2", "VISA Refnum in"=w225) -> ("error out"=w230:errorcluster, "read buffer"=w203:string, "VISA Refnum out"=w231:refnum<visa-resource-name>)  [unwired: 6 in]
            "read buffer 13" <- w203
            n93 = call "Hex to Float.vi"("read buffer in"=w203) -> ("Floating Point"=w179:sgl)  [unwired: 9 in, 1 out]
            "Torque_Ref_readings" <- w179
            n94 = Build Array(w258, w229, w187, w259, w277, w276, w275, w274, w273, w184, w208, w221, w219, w217, w215, w213, w179) -> (w272:dbl[])
            n95 = Array To Spreadsheet String(array=w272, 3:"%f" ("format string")) -> (spreadsheet string=w266:string)  [unwired: 1 in]
            n96 = call "Hex to Float.vi"("read buffer in"=w227) -> ("Floating Point"=→"Speed Reference":sgl)  [unwired: 9 in, 1 out]
            n97 = Write to Text File(file (use dialog)=w270, text=w266, error in=w269) -> (refnum out=w268:refnum<file>, error out=w267:errorcluster)  [unwired: 1 in, 1 out]
          }
        }
        n98 = Wait Until Next ms Multiple(millisecond multiple=u32 1000 ("milliseconds to wait")) -> ()  [unwired: 1 out]
        n99 = Or(x=w168, y="Finish session(Def:Off/False)") -> (x .or. y?=w167:bool)
      }
    }
  }
  n100 = Close File(refnum=w68, error in=w67) -> ()  [unwired: 2 out]
  n101 = case shown="\"Alarm Reset\"" "Enum" {
    tunnel: w69 -> [w290 w295 w299 w318 w362]
    tunnel: w76 -> [w289 w296 w300 w319 w363]
    tunnel: [w288 w293 w303 w313 w364] -> w75
    tunnel: [w287 w294 w304 w316 w365] -> w74
    tunnel: w7 -> [w286 w291 w298 w310 w321]
    tunnel: w6 -> [w285 w292 w297 w309 w322]
    tunnel: [w286 w291 w298 w306 w321] -> w4
    tunnel: [w285 w292 w297 w305 w322] -> w5
    frame "Alarm Reset" {
      n102 = call "Alarm Reset.vi"("error in (no error)"=w290, "VISA Refnum in"=w289) -> ("error out"=w288:errorcluster, "VISA Refnum out"=w287:refnum<visa-resource-name>)  [unwired: 7 in, 1 out]
    }
    frame "Write Save Command" {
      n103 = call "Write Save.vi"("error in (no error)"=w295, "VISA Refnum in"=w296) -> ("error out"=w293:errorcluster, "VISA Refnum out"=w294:refnum<visa-resource-name>)  [unwired: 7 in, 1 out]
    }
    frame "Drive Reset" {
      n104 = call "Write Save.vi"("error in (no error)"=w299, "VISA Refnum in"=w300) -> ("error out"=w301:errorcluster, "VISA Refnum out"=w302:refnum<visa-resource-name>)  [unwired: 7 in, 1 out]
      n105 = call "Drive Reset.vi"("error in (no error)"=w301, "VISA Refnum in"=w302) -> ("error out"=w303:errorcluster, "VISA Refnum out"=w304:refnum<visa-resource-name>)  [unwired: 7 in, 1 out]
    }
    frame "Default" {
      # "This case writes \"0\" to both rpm and torque registers\n to both inverters with the address of 01, 02."
      n106 = VISA Write(VISA resource name=w319, write buffer="\u0002\u0010RÏ\u0000\u0002\u0004\u0000\u0000\u0000\u0000U˜", error in (no error)=w318) -> (VISA resource name out=w315:refnum<visa-resource-name>, error out=w314:errorcluster)  [unwired: 1 out]
      n107 = VISA Write(VISA resource name=w310, write buffer="\u0001\u0010Uï\u0000\u0002\u0004\u0000\u0000\u0000\u0000~ô", error in (no error)=w309) -> (VISA resource name out=w308:refnum<visa-resource-name>, error out=w307:errorcluster)  [unwired: 1 out]
      n108 = VISA Write(VISA resource name=w315, write buffer="\u0002\u0010Uï\u0000\u0002\u0004\u0000\u0000\u0000\u0000q°", error in (no error)=w314) -> (VISA resource name out=w316:refnum<visa-resource-name>, error out=w313:errorcluster)  [unwired: 1 out]
      n109 = VISA Write(VISA resource name=w308, write buffer="\u0001\u0010RÏ\u0000\u0002\u0004\u0000\u0000\u0000\u0000ZÜ", error in (no error)=w307) -> (VISA resource name out=w306:refnum<visa-resource-name>, error out=w305:errorcluster)  [unwired: 1 out]
    }
    frame "Single Signal Trials" {
      n110 = VISA Flush I/O Buffer(VISA resource name=w363, error in (no error)=w362) -> (VISA resource name out=w344:refnum<visa-resource-name>, error out=w345:errorcluster)  [unwired: 1 in]
      n111 = VISA Write(VISA resource name=w344, write buffer="write buffer", error in (no error)=w345) -> (VISA resource name out=w347:refnum<visa-resource-name>, error out=w346:errorcluster)  [unwired: 1 out]
      n112 = VISA Read(VISA resource name=w347, byte count=u32 8, error in (no error)=w346) -> (VISA resource name out=w343:refnum<visa-resource-name>, read buffer=w348:string, error out=w342:errorcluster)  [unwired: 1 out]
      "Answer to Write Command" <- w348
      n113 = call "Hex to Float.vi"("read buffer in"=w348) -> ()  [unwired: 9 in, 2 out]
      n114 = VISA Write(VISA resource name=w343, write buffer="write buffer 2", error in (no error)=w342) -> (VISA resource name out=w353:refnum<visa-resource-name>, error out=w354:errorcluster)  [unwired: 1 out]
      n115 = VISA Read(VISA resource name=w353, byte count=u32 9, error in (no error)=w354) -> (VISA resource name out=w339:refnum<visa-resource-name>, read buffer=w351:string, error out=w338:errorcluster)  [unwired: 1 out]
      "Speed Ref in 21200" <- w351
      n116 = call "Hex to Float.vi"("read buffer in"=w351) -> ("Floating Point"=→"Floating Point 3":sgl)  [unwired: 9 in, 1 out]
      n117 = VISA Write(VISA resource name=w339, write buffer="write buffer 4", error in (no error)=w338) -> (VISA resource name out=w337:refnum<visa-resource-name>, error out=w336:errorcluster)  [unwired: 1 out]
      n118 = VISA Read(VISA resource name=w337, byte count=u32 9, error in (no error)=w336) -> (VISA resource name out=w331:refnum<visa-resource-name>, read buffer=w327:string, error out=w332:errorcluster)  [unwired: 1 out]
      "Speed Ref in 21201" <- w327
      n119 = call "Hex to Float.vi"("read buffer in"=w327) -> ("Floating Point"=→"Floating Point 4":sgl)  [unwired: 9 in, 1 out]
      n120 = VISA Write(VISA resource name=w331, write buffer="write buffer 5", error in (no error)=w332) -> (VISA resource name out=w334:refnum<visa-resource-name>, error out=w333:errorcluster)  [unwired: 1 out]
      n121 = VISA Read(VISA resource name=w334, byte count=u32 9, error in (no error)=w333) -> (VISA resource name out=w329:refnum<visa-resource-name>, read buffer=w323:string, error out=w330:errorcluster)  [unwired: 1 out]
      "Speed Ref in 21201" <- w323
      n122 = call "Hex to Float.vi"("read buffer in"=w323) -> ("Floating Point"=→"Floating Point 5":sgl)  [unwired: 9 in, 1 out]
      n123 = VISA Write(VISA resource name=w329, write buffer="write buffer 3", error in (no error)=w330) -> (VISA resource name out=w359:refnum<visa-resource-name>, error out=w360:errorcluster)  [unwired: 1 out]
      n124 = VISA Read(VISA resource name=w359, byte count=u32 9, error in (no error)=w360) -> (VISA resource name out=w365:refnum<visa-resource-name>, read buffer=w358:string, error out=w364:errorcluster)  [unwired: 1 out]
      "Speed Ref in Monitor" <- w358
      n125 = call "Hex to Float.vi"("read buffer in"=w358) -> ("Floating Point"=→"Floating Point 2":sgl)  [unwired: 9 in, 1 out]
    }
  }
  n126 = VISA Close(VISA resource name=w74, error in (no error)=w75) -> (error out=w3:errorcluster)
  n127 = VISA Close(VISA resource name=w4, error in (no error)=w5) -> (error out=w2:errorcluster)
  n128 = call "Error Fork Stacker.vi"("Error Fork B"=w2, "Error Fork A"=w3) -> ("Error Out"=→"Error Out":errorcluster)  [unwired: 2 in]
